vi "Read CommandQ.vi"(11 "Constellation Command Handler in":refnum<class "Constellation Command Handler.lvclass">) -> (2 "CommandQ":refnum<queue>, 3 "Constellation Command Handler out":refnum<class "Constellation Command Handler.lvclass">)   [LabVIEW 2023, in "VectoScratch.lvlib" / "Constellation Command Handler.lvclass"]
uses:
  Constellation Command Handler.lvclass
  Constellation Command Handler.lvclass/Constellation Command Handler.ctl
  Vecto/proto/ConstellationCommand/Data.ctl
  Vecto/proto/ConstellationCommand/ConstellationCommand.lvlib
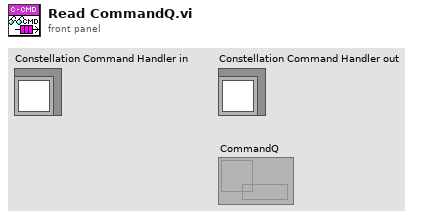
[diagram p1: front panel]
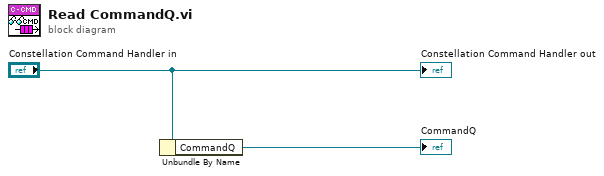
[diagram p0: block diagram]
diagram:
  n1 = Unbundle By Name("Constellation Command Handler in") -> ("CommandQ"=→"CommandQ":refnum<queue>)
  "Constellation Command Handler out" <- "Constellation Command Handler in"
